vi "Remote Time Check Send Init and Final Sync.vi"(6 "Timeout (5000 ms)":dbl=5000.0, 8 "error in (no error)":errorcluster, 11 "connection ID":refnum<k5>) -> (0 "error out":errorcluster, 3 "connection ID out":refnum<k5>)   [LabVIEW 2010, in "Core SubVIs.lvlib"]
uses:
  Core SubVIs.lvlib
  Matlab API/Matlab API.lvlib
panel:
  out "hammer communication":errorcluster
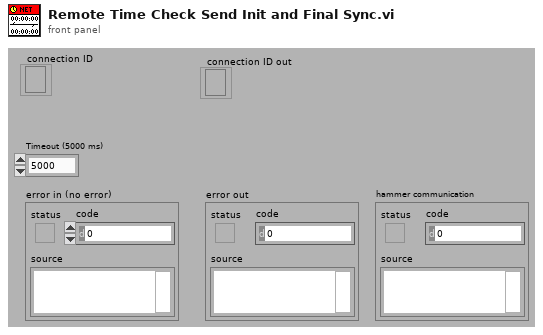
[diagram p1: front panel]
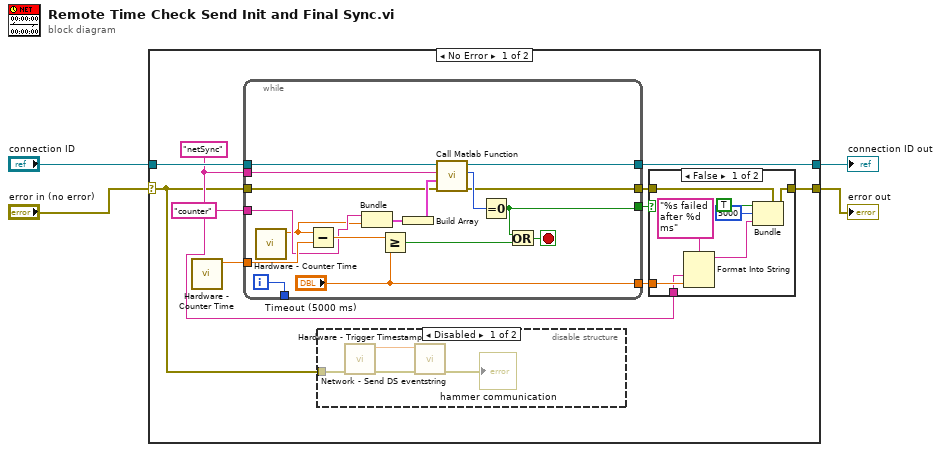
[diagram p0: block diagram]
diagram:
  n1 = case shown="No Error" "error in (no error)" {
    selector: "error in (no error)" -> [w5 w45]
    tunnel: [w14 w46] -> w4
    tunnel: "connection ID" -> [w13 w46]
    tunnel: [w10 w45] -> w2
    frame No Error {
      w7 = "netSync"
      n2 = call "Hardware - Counter Time.vi"() -> ("Timer Value (ms)"=w8:dbl)  [unwired: 3 in, 8 out]
      n3 = while {
        tunnel: w13 -> [w37]
        tunnel: w5 -> [w29]
        tunnel: [w28] -> w11
        tunnel: [w30] -> w14
        tunnel: w7 -> [w36]
        tunnel: w8 -> [w44]
        tunnel: [w32] -> w12
        tunnel: ["Timeout (5000 ms)"] -> w9
        tunnel: [w39] -> _
        tunnel: "counter" -> [w38]
        i -> [w39]
        stop <- w41 stop-if-true
        n4 = call "Hardware - Counter Time.vi"() -> ("Timer Value (ms)"=w35:dbl)  [unwired: 3 in, 8 out]
        n5 = Subtract(x=w35, y=w44) -> (x-y=w43:dbl)
        n6 = Bundle(w38, "Timer Value (ms)"=w35) -> (w34:cluster{string, "Timer Value (ms)":dbl})  [unwired: 1 out]
        n7 = Greater Or Equal?(x=w43, y="Timeout (5000 ms)") -> (x >= y?=w42:bool)
        n8 = Build Array(w34) -> (w33:cluster{string, "Timer Value (ms)":dbl}[])
        n9 = call "Call Matlab Function.vi"("error in (no error)"=w29, "Matlab Param Array"=w33, "Function name"=w36, "TCP Network Connection Refnum"=w37) -> ("error out"=w28:errorcluster, "Return value I32"=w31:i32, "connection ID out"=w30:refnum<k5>)  [unwired: 5 out]
        n10 = Equal To 0?(x=w31) -> (x = 0?=w32:bool)
        n11 = Or(x=w32, y=w42) -> (x .or. y?=w41:bool)
      }
      n12 = disable-structure shown="Disabled" {
        disable-tunnel: w5 -> [w18 _]
        frame Disabled {
          n13 = call "Hardware - Trigger Timestamp.vi"("error in (no error)"=w18) -> ("error out"=w17:errorcluster, "Timer Value (ms)"=w16:dbl)  [unwired: 9 out]
          n14 = call "Network - Send DS eventstring.vi"("error in"=w17, "Numeric"=w16) -> ("error out"=→"hammer communication":errorcluster)  [unwired: 1 in, 8 out]
        }
        frame Enabled {
        }
      }
      n15 = case shown="False" w12 {
        tunnel: w11 -> [w26 w27]
        tunnel: [w25 w27] -> w10
        tunnel: w9 -> [w22 _]
        tunnel: w7 -> [w21 _]
        frame False {
          n16 = Format Into String(format string="%s failed after %d ms", w21, w22) -> (resulting string=w19:string)  [unwired: 2 in, 1 out]
          n17 = Bundle(cluster=w26, "status"=TRUE, "code"=5000, "source"=w19) -> (w25:errorcluster)
        }
        frame True {
        }
      }
    }
    frame Error {
    }
  }
  "error out" <- w2
  "connection ID out" <- w4
